vi "SMF_monitor_V2.0.vi"() -> ()   [LabVIEW 2017]
uses:
  <vilib>/Utility/file.llb/Write Delimited Spreadsheet (string).vi
panel:
  out "Counter":u32
  in  "Tab Control":enum32{"Settings", "Control"}(tab)
  in  "Axis orientation":u16(ring) items=["+x", "-x", "+y", "-y", "+z", "-z", "Reference Test"]
  in  "Test type":u16(ring) items=["Final", "INITIAL", "PASSIVE", "ACTIVE"]
  in  "SMP2 meter":refnum<visa-resource-name>
  in  "Power supply":refnum<visa-resource-name>
  in  "Coil distance":u16(ring) items=["Coil distance=520", "Coil distance=230"]
  in  "Record Button":bool
  out "Voltage":dbl[unit] format="%#_g V"
  in  "stop":bool
  out "Current":dbl[unit] format="%#_g (A)"
  out "Field magnitude":dbl format="%#_g mT"
  in  "Switching off stage":bool
  out "Power off":bool
  out "Desired Current(A)":dbl format="%#_g A"
  out "OutputCurrent":dbl[unit] format="%#_g A"
  in  "Tab Control 2":enum32{"M. Field Control", "Current control"}(tab)
  in  "Desired_M_Field":dbl format="%#_g mT"
  in  "Apply M.Field":bool
  in  "Zero mT M.Field":bool
  in  "Zero M.Field":dbl format="%#_g A"
  out "Sample time":u32
  out "PSU":bool
  out "XY Graph":cluster{dbl[], "array":dbl[]}[](graph)
  # "Gaph Legend"
  # "Conections"
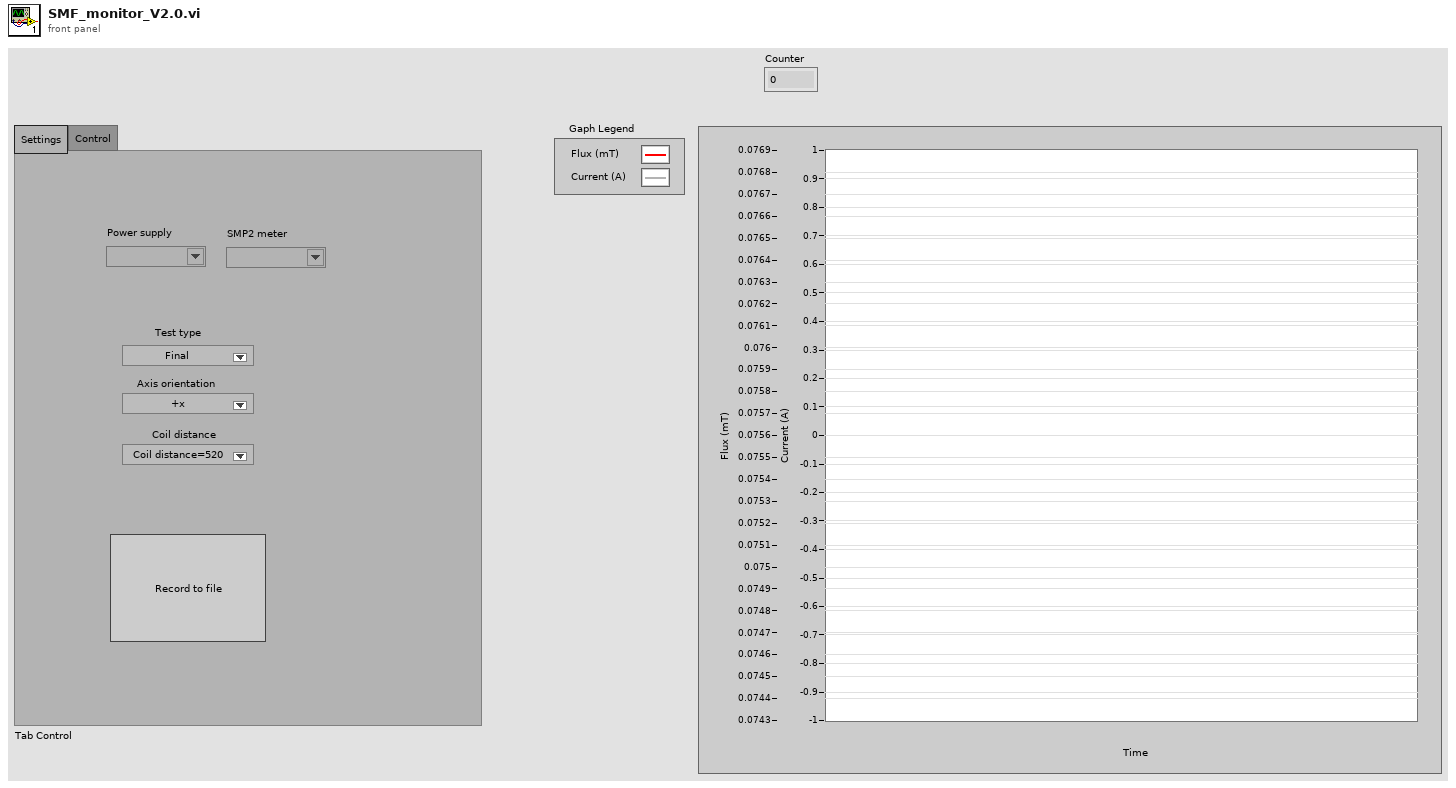
[diagram p1: front panel]
types:
  T1 = enum8{"Enabled", "Disabled", "Disabled and Grayed Out"}
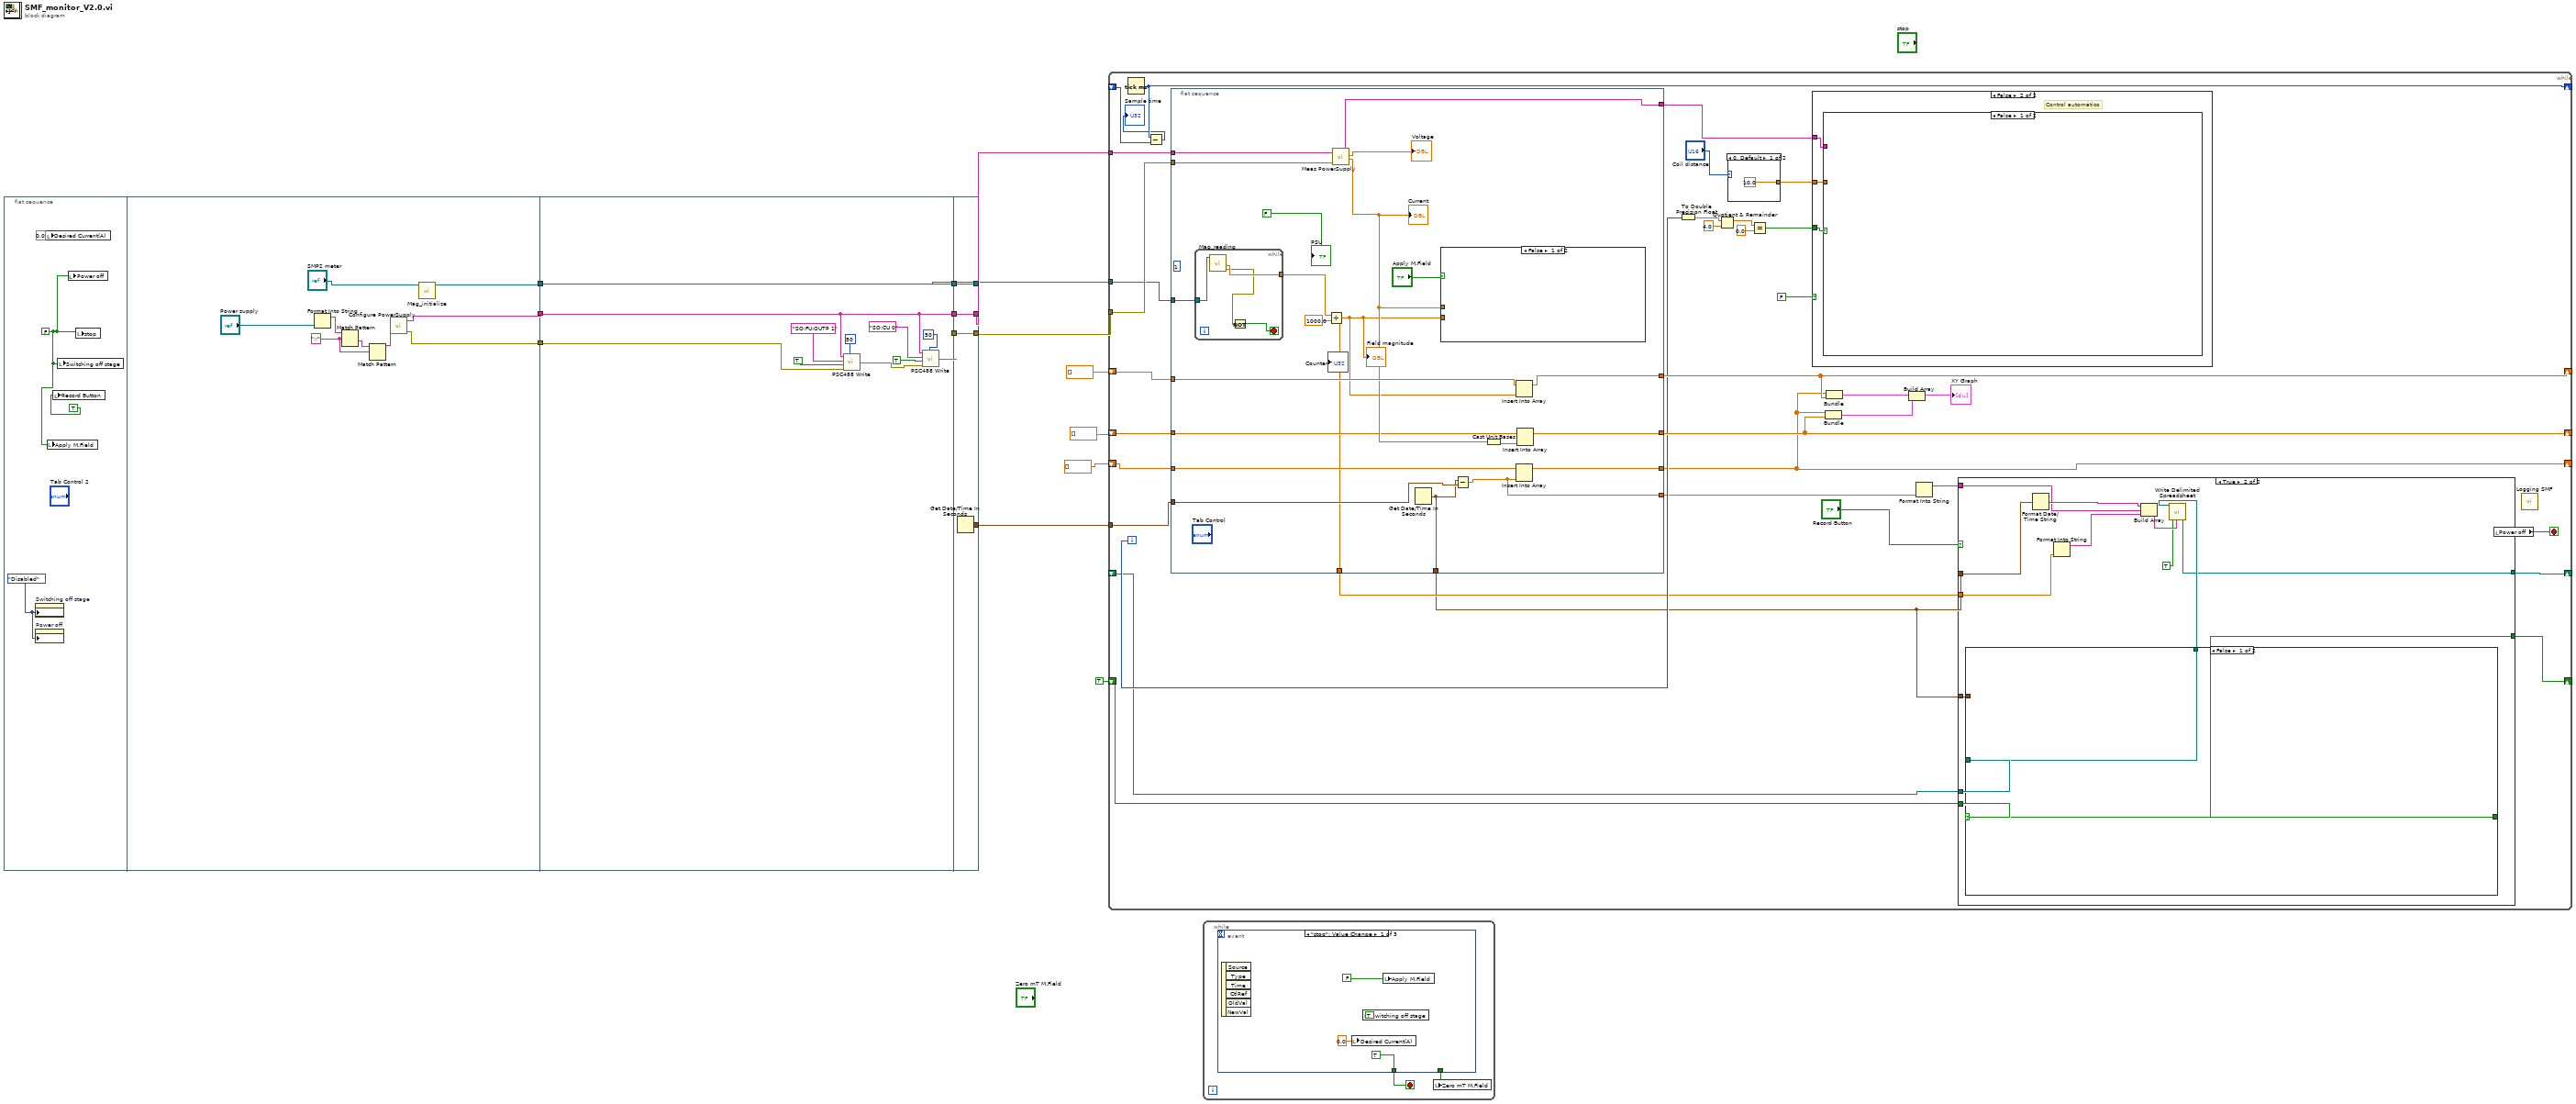
[diagram p0: block diagram]
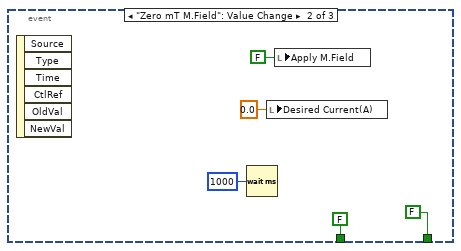
[diagram p2: hidden frame]
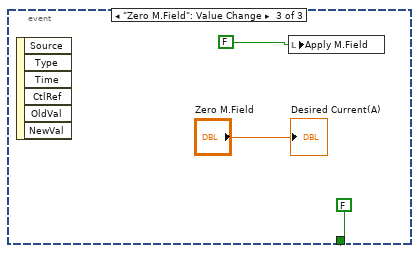
[diagram p3: hidden frame]
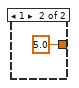
[diagram p4: hidden frame]
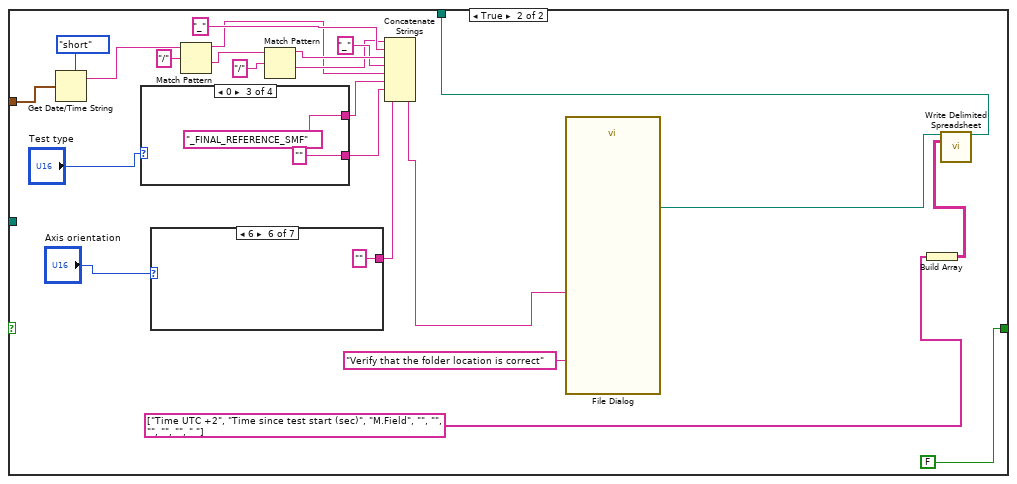
[diagram p6: hidden frame]
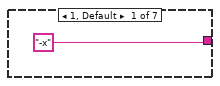
[diagram p7: hidden frame]
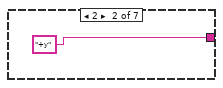
[diagram p8: hidden frame]
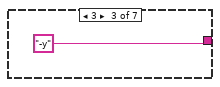
[diagram p9: hidden frame]
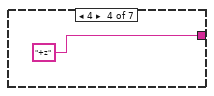
[diagram p10: hidden frame]
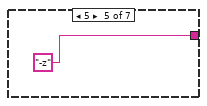
[diagram p11: hidden frame]
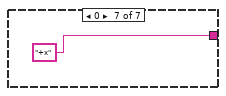
[diagram p12: hidden frame]
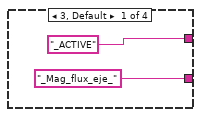
[diagram p13: hidden frame]
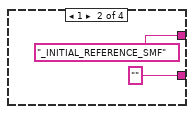
[diagram p14: hidden frame]
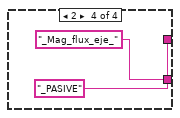
[diagram p15: hidden frame]
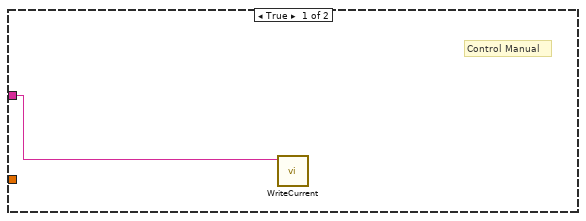
[diagram p16: hidden frame]
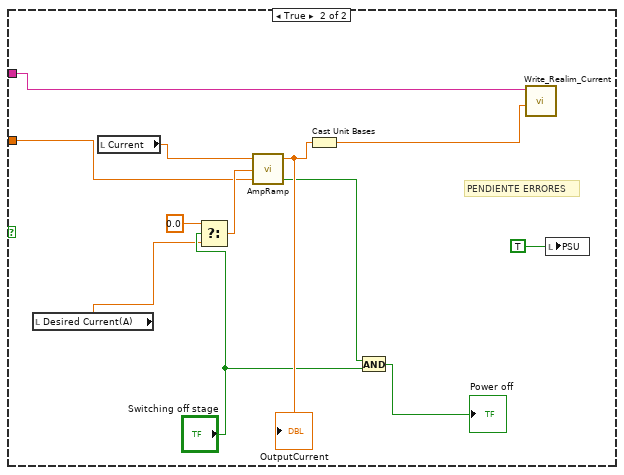
[diagram p17: hidden frame]
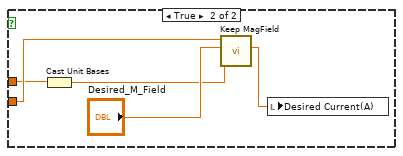
[diagram p18: hidden frame]
diagram:
  n1 = flat-sequence {
    tunnel: [w25] -> w14
    tunnel: [w27] -> w13
    tunnel: [w26] -> w11
    tunnel: w11 -> [w33]
    tunnel: w13 -> [w37]
    tunnel: w14 -> [w38]
    tunnel: [w38] -> w4
    tunnel: [w28] -> w3
    tunnel: [w33] -> w2
    tunnel: [w40] -> w10
    tunnel: [w41] -> w12
    tunnel: [w42] -> w9
    tunnel: w4 -> [w42]
    tunnel: w3 -> [w41]
    tunnel: w2 -> [w40]
    tunnel: [w39] -> w1
    frame #0 {
      w17 = T1."Disabled" ("Disabled")
      w18 = FALSE ("stop")
      n2 = property on="Switching off stage" class="Bool (strict)"("DisabledEnum"=w17) -> ()  [unwired: 2 in, 2 out]
      n3 = property on="Power off" class="Bool (strict)"("DisabledEnum"=w17) -> ()  [unwired: 2 in, 2 out]
      n4 = local write "Desired Current(A)"(0.0 ("Desired Current")) -> ()
      n5 = local write "Apply M.Field"(w18) -> ()
      n6 = local write "Record Button"(TRUE ("Record Button")) -> ()
      n7 = local write "Switching off stage"(w18) -> ()
      n8 = local write "Power off"(w18) -> ()
      n9 = local write "stop"(w18) -> ()
    }
    frame #1 {
      w22 = "::" ("regular expression")
      n10 = Format Into String("Power supply") -> (resulting string=w24:string)  [unwired: 3 in, 1 out]
      n11 = Match Pattern(string=w24, regular expression=w22) -> (after substring=w23:string)  [unwired: 1 in, 3 out]
      n12 = Match Pattern(string=w23, regular expression=w22) -> (before substring=w21:string)  [unwired: 1 in, 3 out]
      n13 = call "Configure PowerSupply.vi"("Address"=w21) -> ("Address Out"=w26:string, "error out"=w27:errorcluster)  [unwired: 6 in]
      n14 = call "Mag_initialize.vi"("VISA resource name"="SMP2 meter") -> ("VISA resource name out"=w25:refnum<visa-resource-name>)  [unwired: 8 in, 1 out]
    }
    frame #2 {
      n15 = call "PSC488 Write.vi"("Address"=w33, "Command"="SO:FU:OUTP 1", "Enable"=TRUE, "error in (no error)"=w37, "Delay after write"=u16 50) -> ("error out"=w29:errorcluster)
      n16 = call "PSC488 Write.vi"("Address"=w33, "Command"="SO:CU 0", "Enable"=TRUE, "error in (no error)"=w29, "Delay after write"=u16 50) -> ("error out"=w28:errorcluster)
    }
    frame #3 {
      n17 = Get Date/Time In Seconds() -> (seconds since 1Jan1904=w39:timestamp)
    }
  }
  n18 = while {
    tunnel: w10 -> [w74]
    tunnel: w12 -> [w78]
    tunnel: w9 -> [w77]
    shift-right: [w70] -> _
    shift-left: dbl[] [] ("array") -> [w76]
    shift-right: [w69] -> _
    shift-left: dbl[] [] ("array") -> [w71]
    shift-right: [w59] -> _
    shift-left: dbl[] [] ("array") -> [w60]
    shift-right: [w57] -> _
    shift-left: TRUE -> [w56]
    shift-right: [w55] -> _
    shift-left: _ -> [w54]
    shift-right: [w53] -> _
    shift-left: _ -> [w52]
    tunnel: w1 -> [w43]
    i -> [w64]
    stop <- w75 stop-if-true
    n19 = Tick Count (ms)() -> (millisecond timer value=w53:u32)
    n20 = Subtract(x=w53, y=w52) -> (x-y=→"Sample time":u32)
    n21 = flat-sequence {
      tunnel: w74 -> [w172]
      tunnel: w78 -> [w171]
      tunnel: w77 -> [w152]
      tunnel: w76 -> [w170]
      tunnel: [w169] -> w70
      tunnel: [w166] -> w73
      tunnel: [w163] -> w59
      tunnel: [w162] -> w69
      tunnel: w71 -> [w161]
      tunnel: w43 -> [w158]
      tunnel: w60 -> [w160]
      tunnel: [w157] -> w46
      tunnel: [w155] -> w50
      tunnel: [w154] -> w45
      frame #0 {
        (unwired) 1
        n22 = while {
          tunnel: [w176] -> w153
          tunnel: w152 -> [w175]
          stop <- w173 stop-if-true
          n23 = call "Mag_reading.vi"("VISA Mag in"=w175) -> ("error out"=w174:errorcluster, "Field magnitude (uT)"=w176:dbl)  [unwired: 8 in, 1 out]
          n24 = Not(x=w174) -> (.not. x?=w173:bool)
        }
        n25 = Divide(x=w153, y=1000.0) -> (x/y=w155:dbl)
        "Field magnitude" <- w155
        n26 = call "Meas PowerSupply.vi"("address string"=w172, "error in (no error)"=w171) -> ("address string 2"=w166:string, "Voltage"=→"Voltage":dbl[unit], "Current"=w164:dbl[unit])  [unwired: 1 in, 1 out]
        "Current" <- w164
        n27 = Get Date/Time In Seconds() -> (seconds since 1Jan1904=w157:timestamp)
        n28 = case shown="False" "Apply M.Field" {
          tunnel: w155 -> [_ w181]
          tunnel: w164 -> [_ w179]
          frame False {
          }
          frame True {
            n29 = Cast Unit Bases(0:w179) -> (2:w177:dbl)  [unwired: 1 in]
            n30 = call "Keep MagField.vi"("Actual_Current"=w177, "Desired_M_Field 2"="Desired_M_Field", "Actual_M_Field"=w181) -> ("Objetive current"=w178:dbl)  [unwired: 8 in]
            n31 = local write "Desired Current(A)"(w178) -> ()
          }
        }
        n32 = Subtract(x=w157, y=w158) -> (x-y=w154:dbl)
        n33 = Cast Unit Bases(0:w164) -> (2:w156:dbl)  [unwired: 1 in]
        n34 = Insert Into Array(array=w170, new element=w155) -> (w169:dbl[])  [unwired: 1 in]
        n35 = Insert Into Array(array=w160, new element=w154) -> (w163:dbl[])  [unwired: 1 in]
        n36 = Insert Into Array(array=w161, new element=w156) -> (w162:dbl[])  [unwired: 1 in]
        "PSU" <- FALSE ("Boolean")
      }
    }
    n37 = To Double Precision Float(number=w64) -> (double precision float=w65:dbl)
    n38 = Quotient & Remainder(x=w65, y=4.0) -> (x-y*floor(x/y)=w62:dbl)  [unwired: 1 out]
    n39 = case shown="0, Default" "Coil distance" {
      tunnel: [10.0 ("Max step A") 5.0 ("Max step A")] -> w48
      frame 0, Default {
      }
      frame 1 {
      }
    }
    n40 = Equal?(x=w62, y=0.0) -> (x = y?=w72:bool)
    n41 = case shown="False" FALSE {
      tunnel: w73 -> [w136 w139]
      tunnel: w72 -> [_ w138]
      tunnel: w48 -> [_ w137]
      frame True {
        # "Control Manual"
        n42 = call "WriteCurrent.vi"("address string in"=w136) -> ()  [unwired: 10 in, 1 out]
      }
      frame False {
        # "Control automático"
        n43 = case shown="False" w138 {
          tunnel: w139 -> [_ w145]
          tunnel: w137 -> [_ w142]
          frame False {
          }
          frame True {
            # "PENDIENTE ERRORES"
            n44 = local read "Desired Current(A)"() -> (w140:dbl)
            n45 = local read "Current"() -> (w149:dbl[unit])
            n46 = Select(t=0.0, s="Switching off stage", f=w140) -> (s? t:f=w147:dbl)
            n47 = call "AmpRamp.vi"("Max step A"=w142, "Desired current (A)"=w147, "Actual Current"=w149) -> ("End Loop"=w150:bool, "OutputCurrent"=w151:dbl[unit])  [unwired: 1 in]
            "OutputCurrent" <- w151
            n48 = Cast Unit Bases(0:w151) -> (2:w144:dbl)  [unwired: 1 in]
            n49 = And(x=w150, y="Switching off stage") -> (x .and. y?=→"Power off":bool)
            n50 = call "Write_Realim_Current.vi"("Objetive Current"=w144, "address string in"=w145) -> ()  [unwired: 8 in, 2 out]
            n51 = local write "PSU"(TRUE ("Boolean")) -> ()
          }
        }
      }
    }
    n52 = Bundle("array"=w59, "array"=w69) -> (w67:cluster{"array":dbl[], "array":dbl[]})  [unwired: 1 in]
    n53 = Bundle("array"=w59, "array"=w70) -> (w68:cluster{"array":dbl[], "array":dbl[]})  [unwired: 1 in]
    n54 = Build Array(w68, w67) -> (→"XY Graph":cluster{"array":dbl[], "array":dbl[]}[])
    n55 = Format Into String(w45) -> (resulting string=w44:string)  [unwired: 3 in, 1 out]
    n56 = case shown="True" "Record Button" {
      tunnel: w46 -> [_ w94]
      tunnel: [w82 w91] -> w57
      tunnel: w56 -> [w82 w92]
      tunnel: [w81 w89] -> w55
      tunnel: w54 -> [w81 w88]
      tunnel: w50 -> [_ w87]
      tunnel: w46 -> [_ w86]
      tunnel: w44 -> [_ w84]
      frame False {
      }
      frame True {
        n57 = case shown="False" w92 {
          selector: w92 -> [w97 _]
          tunnel: [w97 FALSE] -> w91
          tunnel: [w96 w117] -> w90
          tunnel: w88 -> [w96 _]
          tunnel: w86 -> [_ w114]
          frame False {
          }
          frame True {
            n58 = Get Date/Time String(date format (0)=enum16{"short", "long", "abbreviated"}."short", seconds (now)=w114) -> (date string=w108:string)  [unwired: 1 in, 1 out]
            n59 = case shown="0" "Test type" {
              tunnel: ["_ACTIVE" "_INITIAL_REFERENCE_SMF" "_FINAL_REFERENCE_SMF" "_PASIVE"] -> w112
              tunnel: ["_Mag_flux_eje_" ("string") "" ("string") "" ("string") "_Mag_flux_eje_" ("string")] -> w101
              frame 3, Default {
              }
              frame 1 {
              }
              frame 0 {
              }
              frame 2 {
              }
            }
            n60 = case shown="6" "Axis orientation" {
              tunnel: ["-x" "+y" "-y" "+z" "-z" "" "+x"] -> w109
              frame 1, Default {
              }
              frame 2 {
              }
              frame 3 {
              }
              frame 4 {
              }
              frame 5 {
              }
              frame 6 {
              }
              frame 0 {
              }
            }
            n61 = Match Pattern(string=w108, regular expression="/") -> (before substring=w99:string, after substring=w105:string)  [unwired: 1 in, 2 out]
            n62 = Match Pattern(string=w105, regular expression="/") -> (before substring=w103:string, after substring=w100:string)  [unwired: 1 in, 2 out]
            n63 = Concatenate Strings(w100, "_" ("string"), w103, "_" ("string"), w99, w112, w101, w109) -> (w115:string)
            n64 = call "File Dialog"("prompt"="Verify that the folder location is correct", "default name"=w115) -> ("selected path"=w116:path)  [unwired: 10 in, 3 out]
            n65 = Build Array(string[] ["Time UTC +2", "Time since test start (sec)", "M.Field", "", "", "", "", "", " "] ("element")) -> (w118:string[][])
            n66 = call-poly <vilib>:"Write Delimited Spreadsheet.vi"("file path (dialog if empty)"=w116, "2D data"=w118) -> ("new file path (Not A Path if cancelled)"=w117:path)  [unwired: 12 in, 1 out]
          }
        }
        n67 = Format Date/Time String(seconds (now)=w94) -> (date/time string=w85:string)  [unwired: 2 in]
        n68 = Format Into String(w87) -> (resulting string=w83:string)  [unwired: 3 in, 1 out]
        n69 = Build Array(w85, w84, w83) -> (w95:string[])
        n70 = call-poly <vilib>:"Write Delimited Spreadsheet.vi"("file path (dialog if empty)"=w90, "1D data"=w95, "append to file? (new file:F)"=TRUE) -> ("new file path (Not A Path if cancelled)"=w89:path)  [unwired: 11 in, 1 out]
      }
    }
    n71 = local read "Power off"() -> (w75:bool)
    n72 = call "Logging SMF.vi"() -> ()  [unwired: 12 in]
  }
  n73 = while {
    stop <- w183 stop-if-true
    n74 = event shown="[0] \"stop\": Value Change" {
      selector: _ -> [_ _ _]
      dyn-events: _ -> [_ _ _]
      timeout: _ -> [_ _ _]
      tunnel: [TRUE FALSE FALSE] -> w183
      tunnel: [_ FALSE ("Zero") _] -> w182
      event "stop": Value Change {
        n75 = event-data() -> ()  [unwired: 1 in, 6 out]
        n76 = local write "Desired Current(A)"(0.0 ("Desired Current(A)")) -> ()
        n77 = local write "Switching off stage"(TRUE ("Soft Off")) -> ()
        n78 = local write "Apply M.Field"(FALSE ("Keep Level")) -> ()
      }
      event "Zero mT M.Field": Value Change {
        n79 = event-data() -> ()  [unwired: 1 in, 6 out]
        n80 = Wait (ms)(milliseconds to wait=u32 1000) -> ()  [unwired: 1 out]
        n81 = local write "Desired Current(A)"(0.0 ("Desired Current(A)")) -> ()
        n82 = local write "Apply M.Field"(FALSE ("Apply M.Field")) -> ()
      }
      event "Zero M.Field": Value Change {
        n83 = event-data() -> ()  [unwired: 1 in, 6 out]
        n84 = local write "Apply M.Field"(FALSE ("Keep Level")) -> ()
        "Desired Current(A)" <- "Zero M.Field"
      }
    }
    n85 = local write "Zero mT M.Field"(w182) -> ()
  }
